vi "Clamp.vi"() -> ()   [LabVIEW 2016]
doc: "This example illustrates the use of the horizontal clamp tool. You can draw a region of inspection that contains at least two edges in the image. The VI measures the distance between the first and last edges."
uses:
  <vilib>/vision/Pattern Matching.llb/IMAQ Curve Parameters.ctl
  <vilib>/vision/Clamp.llb/Edge Polarity Type.ctl
  <vilib>/vision/NI_Vision_Development_Module.lvlib
panel:
  in  "Distance Type":u16(ring) items=["Horizontal Max", "Clamp Max"]
  out "Distance":sgl
  out "Image":T1(plugin-control)
  in  "Stop":bool
  # "Instructions:\n1. Run the VI.\n2. Draw a Region of Interest in the image containing at least 2 edges to calculate the maximum horizontal distance.\n3. Change the Distance"
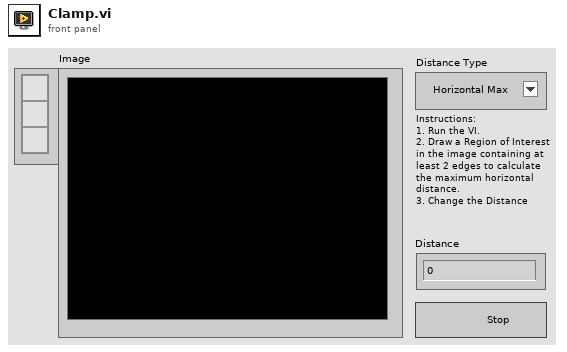
[diagram p1: front panel]
types:
  T1 = typedef "IMAQ Image.ctl" = refnum<image>
  T2 = typedef "IMAQ Rectangle" = cluster{"Left":i32, "Top":i32, "Right":i32, "Bottom":i32, "Rotation":dbl}
  T3 = typedef "ROI Descriptor" = cluster{"Global Rectangle":i32[], "Contours":cluster{"ID":enum32{"External", "Internal"}, "Type":u32, "Coordinates":i32[]}[]}
  T4 = cluster{"Global Rectangle":i32[], "Contours":cluster{"Contour Type":u32, "ROI Type":u32, "Points":i32[]}[]}
  T5 = cluster{"Contrast":i32, "Filter width":i32, "Steepness":i32, "Subsampling Ratio":u32, "Show Search Area":bool, "Show Search Lines":bool, "Show Edges Found":bool, "Show Result":bool}
  T6 = typedef "Edge Polarity Type.ctl" = u32
  T7 = cluster{"Angle Range (+/-)":dbl, "Edge Polarity":cluster{"Start":T6, "End":T6}}
  T8 = typedef "IMAQ Curve Parameters.ctl" = cluster{"Extraction Mode":u32, "Edge Threshold":i32, "Edge Filter Size":u32, "Min Length":i32, "Row Search Step Size":i32, "Col Search Step Size":i32, "Max Endpoint Gap":i32, "Closed":bool, "Subpixel":bool}
  T9 = cluster{"Distance (Pixels)":dbl, "Distance (Real World)":dbl, "Angle (Absolute)":dbl, "Angle (Relative)":dbl}
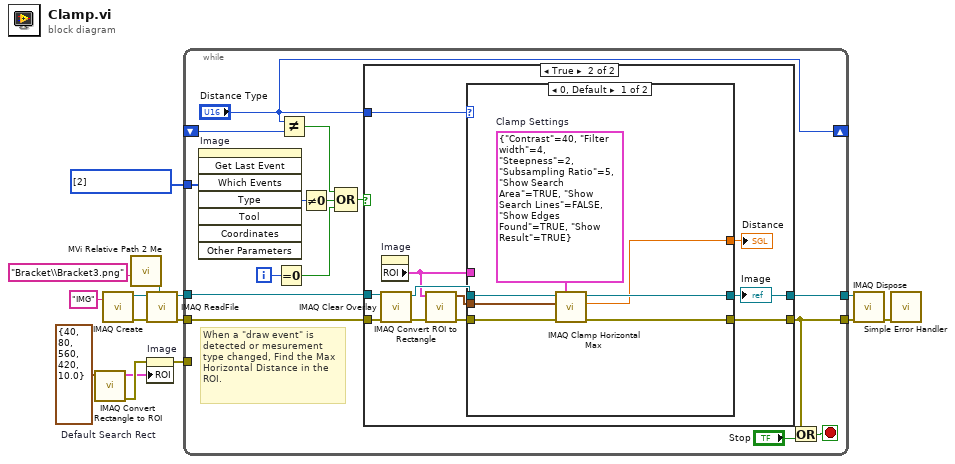
[diagram p0: block diagram]
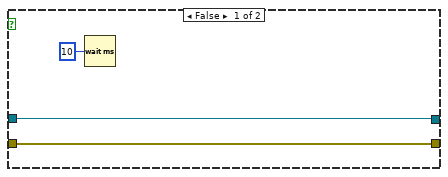
[diagram p2: hidden frame]
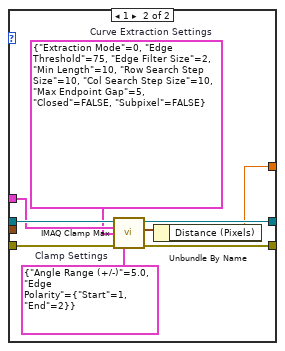
[diagram p3: hidden frame]
diagram:
  w7 = i32[] [2] items=["No  event", "Click event", "Draw event", "Move event", "Size event", "Scroll event", "Activate event", "Close event", "Double click event"] ("Events list (all)")
  w6 = T2 {"Left"=40, "Top"=80, "Right"=560, "Bottom"=420, "Rotation"=10.0}  # Default Search Rect
  n1 = call "IMAQ Convert Rectangle to ROI"("Rectangle"=w6) -> ("error out"=w5:errorcluster, "ROI Descriptor"=w4:T3)  [unwired: 8 in]
  n2 = call "IMAQ Create"("Image Name"="IMG") -> ("Src"=w14:T1, "error out"=w13:errorcluster)  [unwired: 4 in]
  n3 = call "MVi Relative Path 2 Me.vi"("Relative Path"="Bracket\\Bracket3.png" ("name or relative path")) -> ("Appended Dir"=w1:path)  [unwired: 5 in, 1 out]
  n4 = call "IMAQ ReadFile"("File Path"=w1, "error in (no error)"=w13, "Image"=w14) -> ("error out"=w8:errorcluster, "Image Out"=w9:T1)  [unwired: 4 in, 3 out]
  n5 = property on="Image" class="ImageControl"(error in=w5, "ROI"=w4) -> (error out=w3:errorcluster)  [unwired: 1 in, 1 out]
  n6 = while {
    tunnel: w9 -> [w30]
    tunnel: [w24] -> w11
    tunnel: [w22] -> w10
    tunnel: w8 -> [w28]
    tunnel: w7 -> [w27]
    tunnel: w3 -> [_]
    shift-right: ["Distance Type"] -> _
    shift-left: _ -> [w21]
    i -> [w26]
    stop <- w23 stop-if-true
    # "When a \"draw event\" is detected or mesurement type changed, Find the Max Horizontal Distance in the ROI."
    n7 = invoke on="Image" class="ImageControl" method="Get Last Event"("Which Events"=w27) -> ("Type"=w29:i32)  [unwired: 7 in, 7 out]
    n8 = Equal To 0?(x=w26) -> (x = 0?=w16:bool)
    n9 = Not Equal?(x="Distance Type", y=w21) -> (x != y?=w18:bool)
    n10 = Not Equal To 0?(x=w29) -> (x != 0?=w17:bool)
    n11 = Compound Arithmetic op=OR(w18, w17, w16) -> (w19:bool)
    n12 = case shown="True" w19 {
      tunnel: w30 -> [w31 w40]
      tunnel: [w32 w43] -> w24
      tunnel: [w31 w34] -> w22
      tunnel: w28 -> [w32 w42]
      tunnel: "Distance Type" -> [_ w36]
      frame False {
        n13 = Wait (ms)(milliseconds to wait=u32 10) -> ()  [unwired: 1 out]
      }
      frame True {
        n14 = call "IMAQ Clear Overlay"("error in (no error)"=w42, "Image"=w40) -> ("error out"=w39:errorcluster, "Image Out"=w44:T1)  [unwired: 8 in]
        n15 = property on="Image" class="ImageControl"() -> ("ROI"=w37:T4)  [unwired: 2 in, 2 out]
        n16 = call "IMAQ Convert ROI to Rectangle"("error in (no error)"=w39, "ROI Descriptor"=w37) -> ("error out"=w38:errorcluster, "Rectangle"=w41:T2)  [unwired: 7 in]
        n17 = case shown="0, Default" w36 {
          tunnel: w44 -> [w51 w60]
          tunnel: [w49 w58] -> w43
          tunnel: [w48 w57] -> w34
          tunnel: w41 -> [w47 _]
          tunnel: w38 -> [w46 w59]
          tunnel: w37 -> [_ w56]
          tunnel: [w45 w52] -> w35
          frame 0, Default {
            w50 = T5 {"Contrast"=40, "Filter width"=4, "Steepness"=2, "Subsampling Ratio"=5, "Show Search Area"=TRUE, "Show Search Lines"=FALSE, "Show Edges Found"=TRUE, "Show Result"=TRUE}  # Clamp Settings
            n18 = call "IMAQ Clamp Horizontal Max"("Settings"=w50, "error in (no error)"=w46, "Rectangle"=w47, "Image"=w51) -> ("error out"=w49:errorcluster, "Distance"=w45:sgl, "Image Out"=w48:T1)  [unwired: 3 in, 2 out]
          }
          frame 1 {
            w54 = T7 {"Angle Range (+/-)"=5.0, "Edge Polarity"={"Start"=1, "End"=2}}  # Clamp Settings
            w55 = T8 {"Extraction Mode"=0, "Edge Threshold"=75, "Edge Filter Size"=2, "Min Length"=10, "Row Search Step Size"=10, "Col Search Step Size"=10, "Max Endpoint Gap"=5, "Closed"=FALSE, "Subpixel"=FALSE}  # Curve Extraction Settings
            n19 = call "IMAQ Clamp Max"("Source Image"=w60, "ROI Descriptor"=w56, "Curve Extraction Settings"=w55, "error in (no error)"=w59, "Clamp Settings"=w54) -> ("Image Out"=w57:T1, "Clamp Results"=w53:T9, "error out"=w58:errorcluster)  [unwired: 5 in, 3 out]
            n20 = Unbundle By Name(w53) -> ("Distance (Pixels)"=w52:dbl)
          }
        }
        "Distance" <- w35
        "Image" <- w34
      }
    }
    n21 = Or(x=w24, y="Stop") -> (x .or. y?=w23:bool)
  }
  n22 = call "IMAQ Dispose"("Image"=w10, "error in (no error)"=w11) -> ("error out"=w15:errorcluster)  [unwired: 4 in]
  n23 = call <vilib>:"Simple Error Handler.vi"("error in (no error)"=w15) -> ()  [unwired: 4 in, 5 out]
